vi "Create from VI.vi"(8 "error in (no error)":errorcluster, 9 "Test Method VI Path":path, 10 "Test Case LVCLass Path":path) -> (0 "error out":errorcluster, 3 "LUnit Test Case Out":refnum<class "LUnit Inheriting Test Case.lvclass">)   [LabVIEW 2020]
uses:
  LUnit Inheriting Test Case.lvclass
  C:/git/astemes-lunit/source/API/LUnit Inheriting Test Case/LUnit Test Case/LUnit Inheriting Test Case.lvclass
  C:/git/astemes-lunit/source/Core/Runnable/Runnable.lvclass
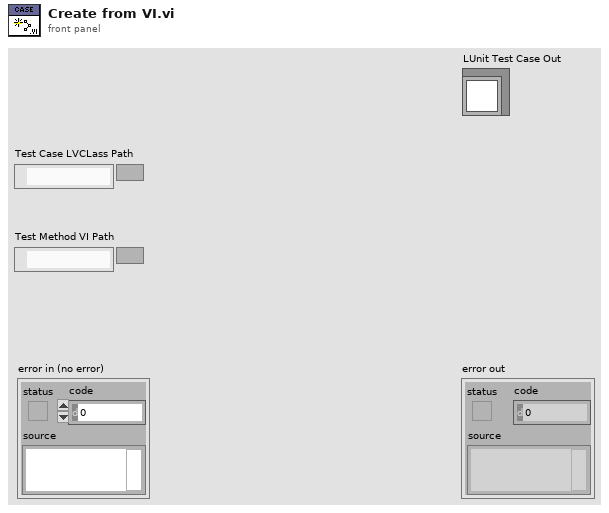
[diagram p1: front panel]
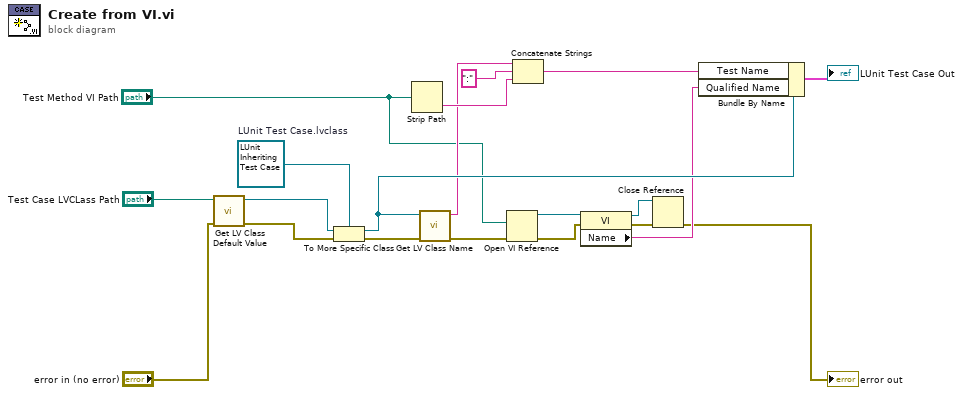
[diagram p0: block diagram]
diagram:
  w16 = refnum<class "LUnit Inheriting Test Case.lvclass"> refnum  # LUnit Test Case.lvclass
  n1 = call <vilib>:"Get LV Class Default Value.vi"("error in (no error)"="error in (no error)", "class path"="Test Case LVCLass Path") -> ("error out"=w18:errorcluster, "object"=w19:refnum<class>)  [unwired: 8 in]
  n2 = To More Specific Class(target class=w16, reference=w19, error in=w18) -> (specific class reference=w12:refnum<class "LUnit Inheriting Test Case.lvclass">, error out=w11:errorcluster)
  n3 = Strip Path(path="Test Method VI Path") -> (name=w14:string)  [unwired: 1 out]
  n4 = call <vilib>:"Get LV Class Name.vi"("error in (no error)"=w11, "object"=w12) -> ("error out"=w2:errorcluster, "class name"=w10:string)  [unwired: 8 in]
  n5 = Open VI Reference(vi path="Test Method VI Path", error in (no error)=w2) -> (vi reference=w7:refnum<vi>, error out=w5:errorcluster)  [unwired: 4 in]
  n6 = Concatenate Strings(w10, ":" ("string"), w14) -> (w9:string)
  n7 = property class="VI"(reference=w7, error in=w5) -> (reference out=w3:refnum<vi>, error out=w4:errorcluster, "Name"=w6:string)
  n8 = Close Reference(reference=w3, error in (no error)=w4) -> (error out=→"error out":errorcluster)
  n9 = Bundle By Name(cluster=w12, "Test Name"=w9, "Qualified Name"=w6) -> (→"LUnit Test Case Out":cluster{})
